vi "Get Last Error.vi"(8 "error in":errorcluster) -> (0 "error out":errorcluster)   [LabVIEW 2019, in "PCANBasic.lvlib" / "Read Event.lvclass"]
uses:
  Read Event.lvclass
  Read Event.lvclass/Read Event.ctl
  PCANBasic.lvlib
panel:
  out "Last Error":u32
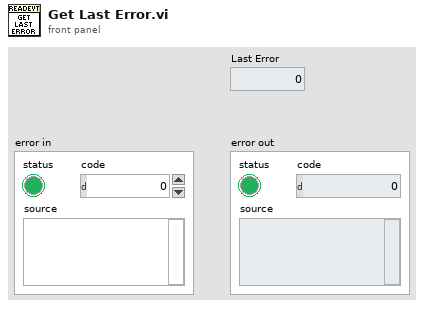
[diagram p1: front panel]
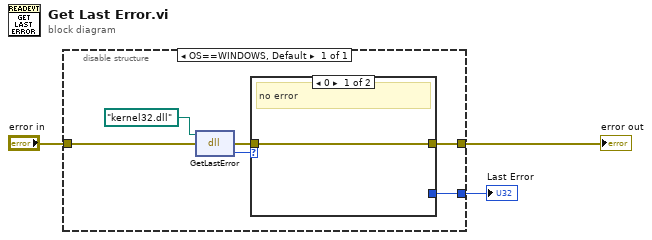
[diagram p0: block diagram]
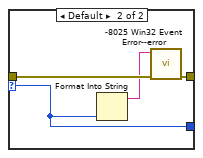
[diagram p2: hidden frame]
diagram:
  n1 = disable-structure shown="OS==WINDOWS, Default" {
    disable-tunnel: "error in" -> [w9]
    disable-tunnel: [w5] -> w2
    disable-tunnel: [w4] -> w1
    frame condition #0 (active) {
      n2 = dll-call lib="?" fn="GetLastError"(path in=path "kernel32.dll", error in=w9) -> (error out=w6:errorcluster, "error"=w7:u32)  [unwired: 1 in, 1 out]
      n3 = case shown="0" w7 {
        selector: w7 -> [_ w11]
        tunnel: w6 -> [w10 w14]
        tunnel: [w10 w12] -> w5
        tunnel: [_ w11] -> w4
        frame 0 {
          # "no error"
        }
        frame Default {
          n4 = Format Into String(w11) -> (resulting string=w13:string)  [unwired: 3 in, 1 out]
          n5 = call "-8025 Win32 Event Error--error.vi"("error in"=w14, "Argument"=w13) -> ("error out"=w12:errorcluster)  [unwired: 8 in, 1 out]
        }
      }
    }
  }
  "error out" <- w2
  "Last Error" <- w1
